vi "Drive PID.vi"(4 "reinitialize? (F)":bool, 5 "coast?":bool, 6 "PID Params":T1={"PID gains"={"proportional gain (Kc)"=1.0, "integral time (Ti, min)"=0.0, "derivative time (Td, min)"=0.0}, "output range"={"output high"=1.0, "output low"=-1.0}}, 7 "Setpoint":dbl, 8 "Max Stop Speed":dbl, 9 "Distance Stop Threshold":dbl, 10 "Current Speed":dbl, 11 "Current Distance":dbl format="%#_13g") -> (0 "Finished":bool, 2 "output":dbl format="%.2f")   [LabVIEW 2013]
uses:
  Common Code/Change Detect Boolean.vi
  <vilib>/addons/control/pid/pid.llb/PID (DBL).vi
  <vilib>/addons/control/pid/NI_PID_pid.lvlib
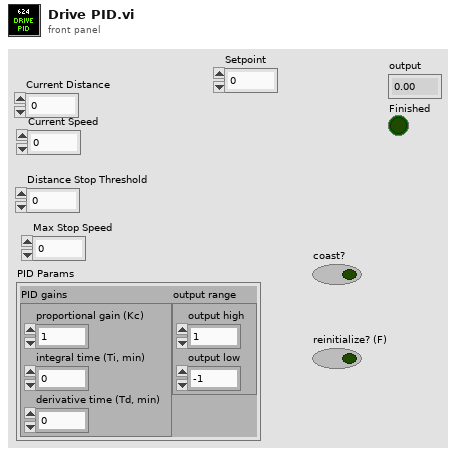
[diagram p1: front panel]
types:
  T1 = cluster{"PID gains":cluster{"proportional gain (Kc)":dbl, "integral time (Ti, min)":dbl, "derivative time (Td, min)":dbl}, "output range":cluster{"output high":dbl, "output low":dbl}}
  T2 = cluster{"proportional gain (Kc)":dbl, "integral time (Ti, min)":dbl, "derivative time (Td, min)":dbl}
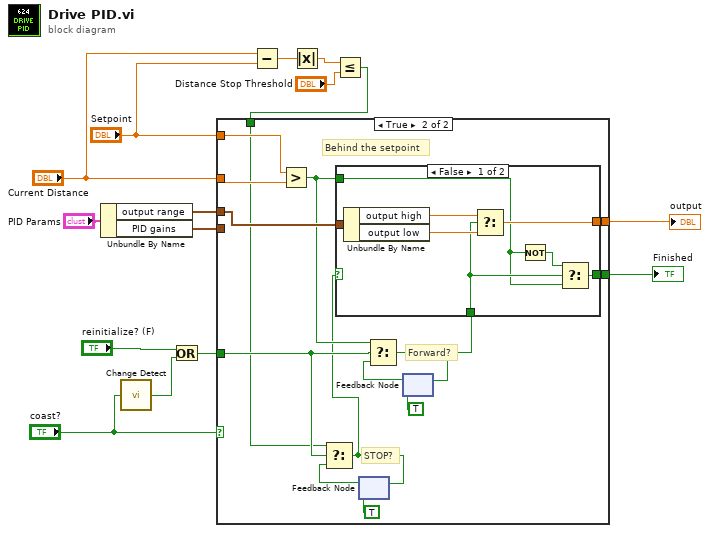
[diagram p0: block diagram]
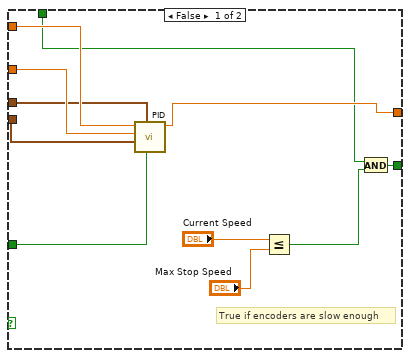
[diagram p2: hidden frame]
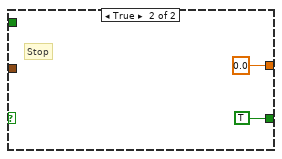
[diagram p3: hidden frame]
diagram:
  n1 = Unbundle By Name("PID Params") -> ("output range"=w12:cluster{"output high":dbl, "output low":dbl}, "PID gains"=w11:T2)
  n2 = call-poly "Change Detect.vi"("In"="coast?") -> ("Changed?"=w3:bool)
  n3 = Or(x="reinitialize? (F)", y=w3) -> (x .or. y?=w1:bool)
  n4 = Subtract(x="Current Distance", y="Setpoint") -> (x-y=w8:dbl)
  n5 = Absolute Value(x=w8) -> (abs(x)=w6:dbl)
  n6 = Less Or Equal?(x=w6, y="Distance Stop Threshold") -> (x <= y?=w5:bool)
  n7 = case shown="True" "coast?" {
    tunnel: w1 -> [w26 w29]
    tunnel: "Current Distance" -> [w25 w33]
    tunnel: "Setpoint" -> [w24 w34]
    tunnel: w12 -> [w21 w40]
    tunnel: w11 -> [w20 _]
    tunnel: [w18 w36] -> w10
    tunnel: [w17 w39] -> w9
    tunnel: w5 -> [w16 w28]
    frame False {
      # "True if encoders are slow enough"
      n8 = call-poly <vilib>:"PID.vi"("reinitialize? (F)"=w26, "output range"=w21, "PID gains"=w20, "process variable"=w25, "setpoint"=w24) -> ("output"=w17:dbl)  [unwired: 5 in, 1 out]
      n9 = Less Or Equal?(x="Current Speed", y="Max Stop Speed") -> (x <= y?=w19:bool)
      n10 = And(x=w16, y=w19) -> (x .and. y?=w18:bool)
    }
    frame True {
      # "STOP?"
      # "Behind the setpoint"
      # "Forward?"
      n11 = Greater?(x=w34, y=w33) -> (0:w32:bool)
      n12 = feedback #1(TRUE) -> (w31:bool)
      n13 = Select(t=w28, s=w29, f=w31) -> (s? t:f=w27:bool)
      n14 = feedback-in #1(w27) -> ()
      n15 = feedback #2(TRUE) -> (w37:bool)
      n16 = Select(t=w32, s=w29, f=w37) -> (s? t:f=w35:bool)
      n17 = case shown="False" w27 {
        tunnel: w40 -> [w48 _]
        tunnel: [w45 0.0 ("output low")] -> w39
        tunnel: [w44 TRUE] -> w36
        tunnel: w35 -> [w43 _]
        tunnel: w32 -> [w41 _]
        frame False {
          n18 = Unbundle By Name(w48) -> ("output high"=w46:dbl, "output low"=w47:dbl)
          n19 = Select(t=w46, s=w43, f=w47) -> (s? t:f=w45:dbl)
          n20 = Not(x=w41) -> (.not. x?=w42:bool)
          n21 = Select(t=w42, s=w43, f=w41) -> (s? t:f=w44:bool)
        }
        frame True {
          # "Stop"
        }
      }
      n22 = feedback-in #2(w35) -> ()
    }
  }
  "Finished" <- w10
  "output" <- w9
